vi "nanocal -- defaut parameter manager -- V1.vi"(6 "parameter key array":T1[](array[typedef]), 7 "action":T2=enum."update", 8 "T":dbl=0.269210160049 format="%#_13g", 9 "internal map":map{T1, dbl[]}(c390), 10 "what":T1, 11 "string Map IN":map{string, map{T1, dbl}}(c390)) -> (0 "internal map OUT":map{T1, dbl[]}(c390), 1 "number":dbl, 2 "temporary map OUT":map{T1, dbl[]}(c390))   [LabVIEW 2021]
uses:
  3-lorentzian-parameters.ctl
  nanocal -- defaut parameter manager action-- V1.ctl
  a0897498-3b9b-9348-9f00-d566c8ac58a9.vi
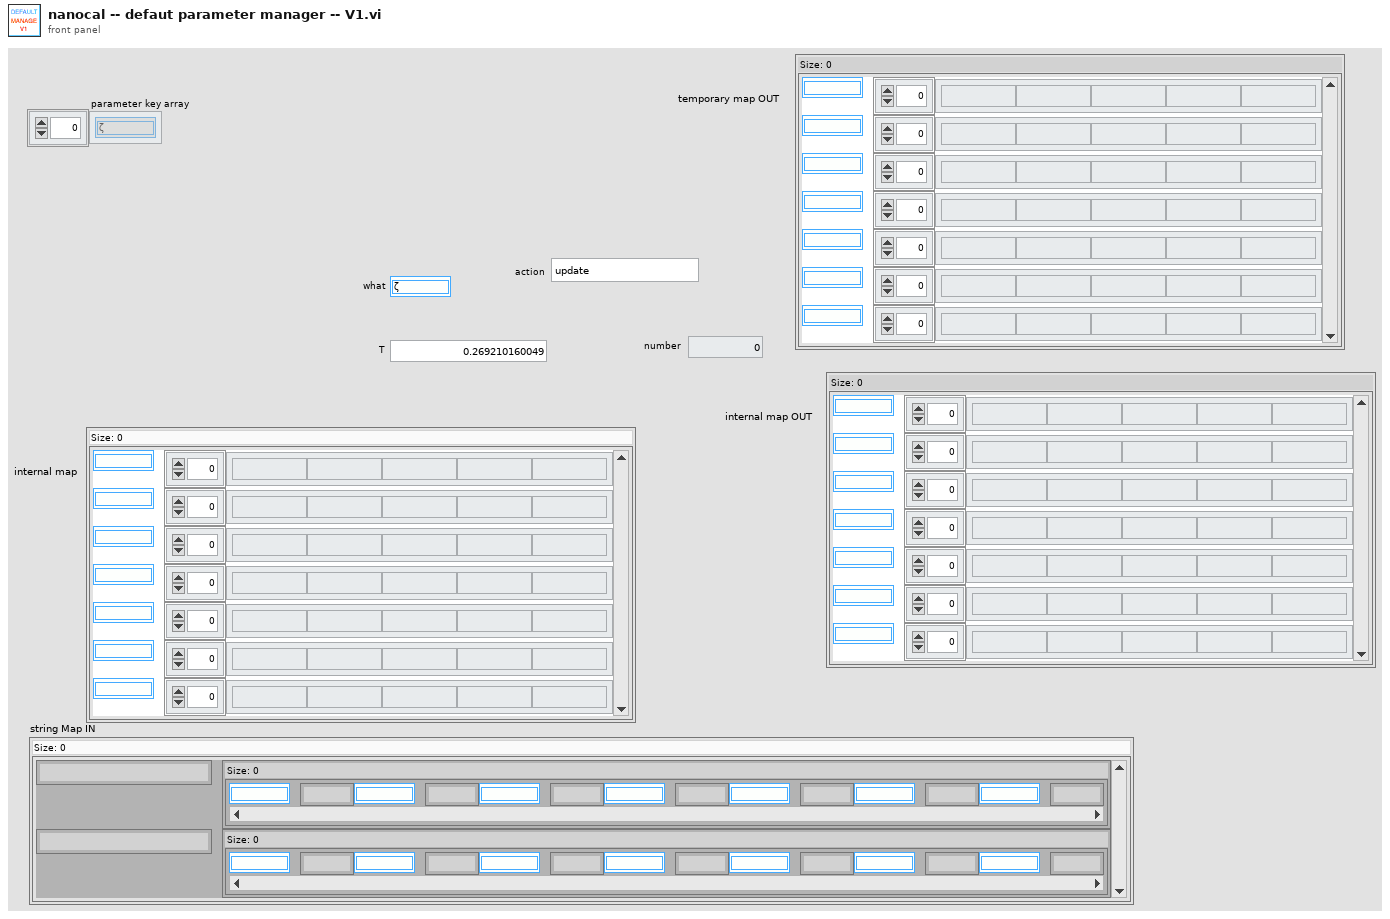
[diagram p1: front panel]
types:
  T1 = typedef "3-lorentzian-parameters.ctl" = enum16{"ζ", "τ1", "τS", "τN", "τC", "κ0", "m1", "m2", "m3", "T (K)", "B (T)", "θ (deg)", "side (S|R)", "set of (B|T)", "Re(offset)", "Im(offset)", "στ1", "στ1-", "στ1+", "στS", "στS-", "στS+", "στN", "στN-", "στN+", "τ11", "τ12", "τ21", "τ22", "τN1", "τN2", "σηlogτ1", "σηlogτS", "σηlogτN", "σlogτ1", "σlogτS", "σlogτN", "σητ1", "σητS", "σητN", "noiseT"}
  T2 = typedef "nanocal -- defaut parameter manager action-- V1.ctl" = enum16{"get logarithmic interp", "update", "get linear interp", "init", "preprocess"}
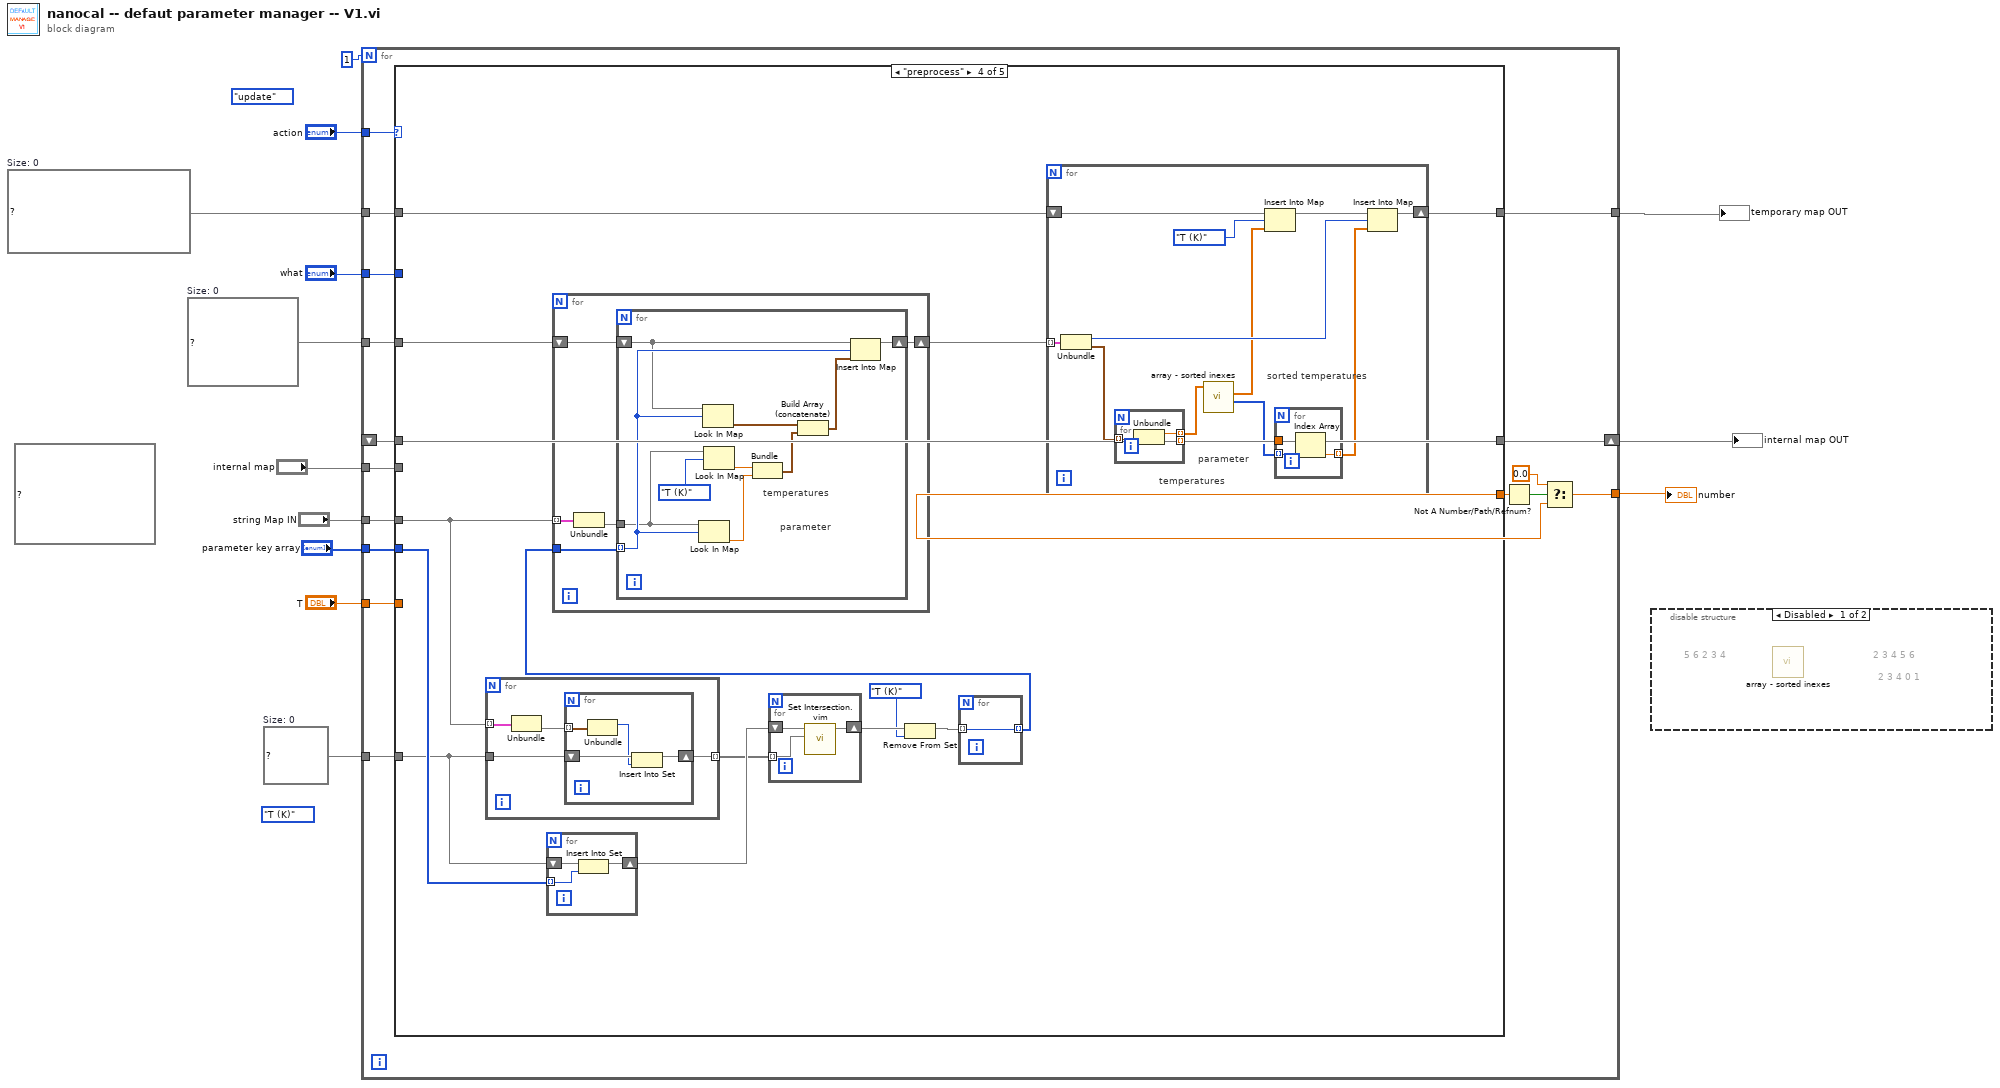
[diagram p0: block diagram]
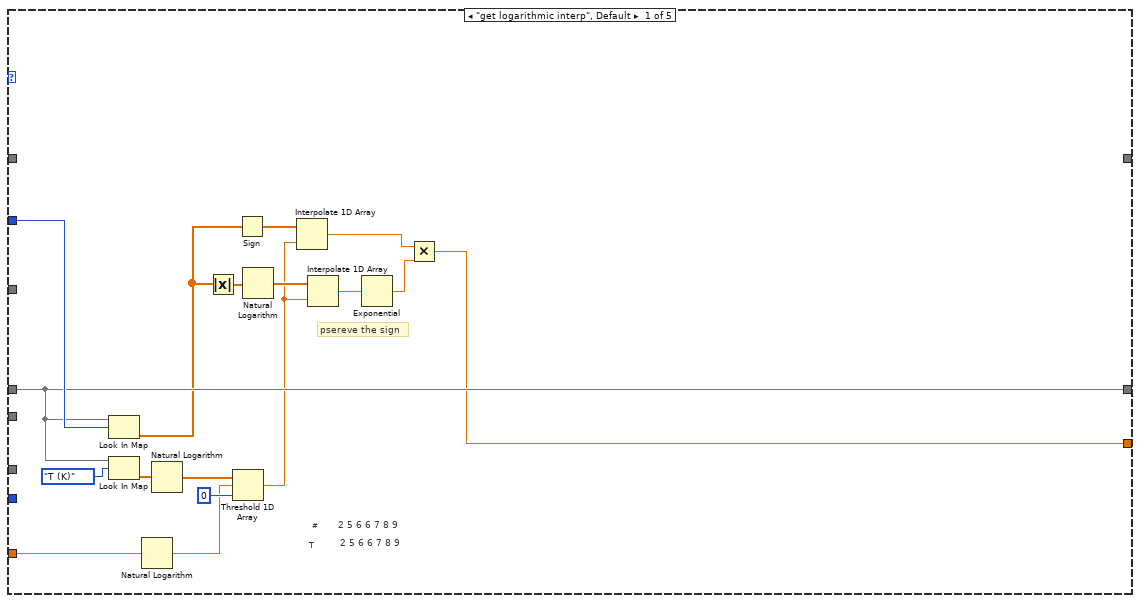
[diagram p3: hidden frame]
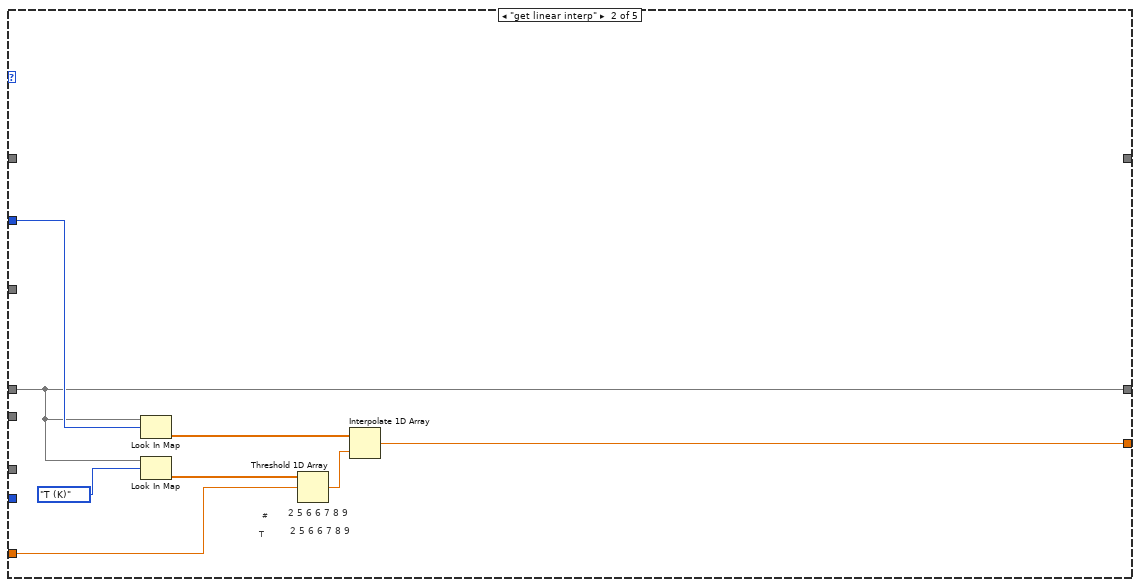
[diagram p4: hidden frame]
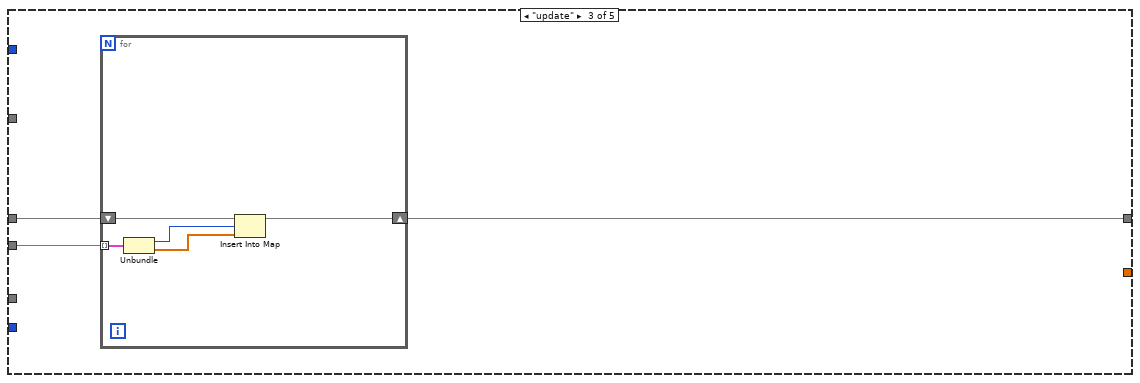
[diagram p5: hidden frame]
diagram:
  (unwired) 3-lorentzian-parameters."T (K)" ("Plost: sweep window")
  w1 = set{T1} {}  # Size: 0
  w2 = map{T1, cluster{"ζ":dbl, "ζ":dbl}[]} {}  # Size: 0
  (unwired) map{string, map{T1, dbl}} {} ("Map OUT")
  (unwired) nanocal_--_defaut_parameter_manager_action--_V1."update" ("action")
  w7 = map{T1, dbl[]} {}  # Size: 0
  n1 = for {
    N: 1 -> [_]
    tunnel: "action" -> [w29]
    shift-right: [w28] -> w3
    shift-left: _ -> [w27]
    tunnel: "internal map" -> [w26]
    tunnel: "what" -> [w25]
    tunnel: "T" -> [w24]
    tunnel: [w22] -> w9
    tunnel: w7 -> [w19]
    tunnel: "string Map IN" -> [w18]
    tunnel: "parameter key array" -> [w17]
    tunnel: [w16] -> w4
    tunnel: w2 -> [w15]
    tunnel: w1 -> [w14]
    n2 = case shown="\"preprocess\"" w29 {
      tunnel: [w44 w52 w55 w76 w125] -> w28
      tunnel: w27 -> [w44 w52 w56 w76 _]
      tunnel: w26 -> [_ _ w57 _ _]
      tunnel: w25 -> [w46 w54 _ _ _]
      tunnel: w24 -> [w38 w51 _ _ _]
      tunnel: [w30 w48 _ _ _] -> w20
      tunnel: w19 -> [_ _ _ w73 w125]
      tunnel: w18 -> [_ _ _ w72 _]
      tunnel: w17 -> [_ _ _ w70 _]
      tunnel: [_ _ _ w74 _] -> w16
      tunnel: w15 -> [_ _ _ w71 _]
      tunnel: w14 -> [_ _ _ w69 _]
      frame "get logarithmic interp", Default {
        # "psereve the sign"
        # "#"
        # "T"
        # "2 5 6 6 7 8 9"
        # "2 5 6 6 7 8 9"
        n3 = Look In Map(map=w44, key=w46) -> (value=w36:dbl[])  [unwired: 1 in, 1 out]
        n4 = Look In Map(map=w44, key=3-lorentzian-parameters."T (K)" ("Plost: sweep window")) -> (value=w43:dbl[])  [unwired: 1 in, 1 out]
        n5 = Natural Logarithm(1:w38) -> (0:w37:dbl)
        n6 = Natural Logarithm(1:w43) -> (0:w42:dbl[])
        n7 = Absolute Value(x=w36) -> (abs(x)=w35:dbl[])
        n8 = Threshold 1D Array(1:0 ("start index (0)"), 2:w37, 3:w42) -> (0:w34:dbl)
        n9 = Sign(1:w36) -> (0:w33:dbl[])
        n10 = Natural Logarithm(1:w35) -> (0:w41:dbl[])
        n11 = Interpolate 1D Array(1:w34, 2:w33) -> (0:w31:dbl)
        n12 = Interpolate 1D Array(1:w34, 2:w41) -> (0:w40:dbl)
        n13 = Exponential(1:w40) -> (0:w32:dbl)
        n14 = Multiply(x=w31, y=w32) -> (x*y=w30:dbl)
      }
      frame "get linear interp" {
        # "#"
        # "T"
        # "2 5 6 6 7 8 9"
        # "2 5 6 6 7 8 9"
        n15 = Look In Map(map=w52, key=w54) -> (value=w49:dbl[])  [unwired: 1 in, 1 out]
        n16 = Look In Map(map=w52, key=3-lorentzian-parameters."T (K)" ("Plost: sweep window")) -> (value=w47:dbl[])  [unwired: 1 in, 1 out]
        n17 = Threshold 1D Array(2:w51, 3:w47) -> (0:w50:dbl)  [unwired: 1 in]
        n18 = Interpolate 1D Array(1:w50, 2:w49) -> (0:w48:dbl)
      }
      frame "update" {
        n19 = for {
          tunnel: w57 -> [w62] mode=indexing
          shift-right: [w60] -> w55
          shift-left: w56 -> [w61]
          n20 = Unbundle(w62) -> ("Plost: sweep window"=w59:T1, w58:dbl[])
          n21 = Insert Into Map(map in=w61, key=w59, value=w58) -> (map out=w60:map{T1, dbl[]})  [unwired: 2 out]
        }
      }
      frame "preprocess" {
        n22 = for {
          tunnel: w72 -> [w87] mode=indexing
          tunnel: w69 -> [w85]
          tunnel: [w84] -> w67 mode=indexing
          n23 = Unbundle(w87) -> ("Map"=w86:map{T1, dbl})  [unwired: 1 out]
          n24 = for {
            tunnel: w86 -> [w91] mode=indexing
            shift-right: [w89] -> w84
            shift-left: w85 -> [w90]
            n25 = Unbundle(w91) -> ("X selector"=w88:T1)  [unwired: 1 out]
            n26 = Insert Into Set(10:w88, 11:w90) -> (3:w89:set{T1})  [unwired: 1 out]
          }
        }
        n27 = for {
          shift-right: [w82] -> w68
          shift-left: w69 -> [w83]
          tunnel: w70 -> [w81] mode=indexing
          n28 = Insert Into Set(10:w81, 11:w83) -> (3:w82:set{T1})  [unwired: 1 out]
        }
        n29 = for {
          shift-right: [w80] -> w66
          shift-left: w68 -> [w79]
          tunnel: w67 -> [w78] mode=indexing
          n30 = call "Set Intersection.vim"("set 2"=w78, "set 1"=w79) -> ("intersection"=w80:set{T1})  [unwired: 9 in]
        }
        n31 = Remove From Set(10:3-lorentzian-parameters."T (K)" ("Plost: sweep window"), 11:w66) -> (3:w64:set{T1})  [unwired: 1 out]
        n32 = for {
          tunnel: w64 -> [w77] mode=indexing
          tunnel: [w77] -> w63 mode=indexing
        }
        n33 = for {
          tunnel: w72 -> [w114] mode=indexing
          tunnel: w63 -> [w113]
          shift-right: [w111] -> w75
          shift-left: w71 -> [w110]
          n34 = Unbundle(w114) -> ("Map"=w112:map{T1, dbl})  [unwired: 1 out]
          n35 = for {
            tunnel: w113 -> [w122] mode=indexing
            tunnel: w112 -> [w121]
            shift-right: [w116] -> w111
            shift-left: w110 -> [w115]
            # "parameter"
            # "temperatures"
            n36 = Look In Map(map=w121, key=w122) -> (value=w118:dbl)  [unwired: 1 in, 1 out]
            n37 = Look In Map(map=w115, key=w122) -> (value=w124:cluster{"ζ":dbl, "ζ":dbl}[])  [unwired: 1 in, 1 out]
            n38 = Look In Map(map=w121, key=3-lorentzian-parameters."T (K)" ("Plost: sweep window")) -> (value=w119:dbl)  [unwired: 1 in, 1 out]
            n39 = Bundle("ζ"=w119, "ζ"=w118) -> (w117:cluster{"ζ":dbl, "ζ":dbl})  [unwired: 1 in]
            n40 = Build Array (concatenate)(w124, w117) -> (w123:cluster{"ζ":dbl, "ζ":dbl}[])
            n41 = Insert Into Map(map in=w115, key=w122, value=w123) -> (map out=w116:map{T1, cluster{"ζ":dbl, "ζ":dbl}[]})  [unwired: 2 out]
          }
        }
        n42 = for {
          tunnel: w75 -> [w103] mode=indexing
          shift-right: [w100] -> w74
          shift-left: w73 -> [w99]
          # "sorted temperatures"
          # "parameter"
          # "temperatures"
          n43 = Unbundle(w103) -> ("Plost: sweep window"=w97:T1, w102:cluster{"ζ":dbl, "ζ":dbl}[])
          n44 = for {
            tunnel: w102 -> [w109] mode=indexing
            tunnel: [w108] -> w101 mode=indexing
            tunnel: [w107] -> w94 mode=indexing
            n45 = Unbundle(w109) -> ("ζ"=w108:dbl, "ζ"=w107:dbl)
          }
          n46 = call "array - sorted inexes.vi"("x"=w101) -> ("index array"=w93:i32[], "sorted array"=w95:dbl[])  [unwired: 9 in]
          n47 = Insert Into Map(map in=w99, key=3-lorentzian-parameters."T (K)", value=w95) -> (map out=w98:map{T1, dbl[]})  [unwired: 2 out]
          n48 = for {
            tunnel: w94 -> [w106]
            tunnel: w93 -> [w105] mode=indexing
            tunnel: [w104] -> w92 mode=indexing
            n49 = Index Array(array=w106, index=w105) -> (element=w104:dbl)
          }
          n50 = Insert Into Map(map in=w98, key=w97, value=w92) -> (map out=w100:map{T1, dbl[]})  [unwired: 2 out]
        }
      }
      frame "init" {
      }
    }
    n51 = Not A Number/Path/Refnum?(number/path/refnum=w20) -> (NaN/Path/Refnum?=w23:bool)
    n52 = Select(t=0.0, s=w23, f=w20) -> (s? t:f=w22:dbl)
  }
  "number" <- w9
  "temporary map OUT" <- w4
  "internal map OUT" <- w3
  n53 = disable-structure shown="Disabled" {
    frame Disabled {
      # "2 3 4 0 1"
      # "2 3 4 5 6"
      # "5 6 2 3 4"
      n54 = call "array - sorted inexes.vi"() -> ()  [unwired: 10 in, 2 out]
    }
    frame Enabled {
    }
  }
